vi "MultiFileGraphChoose.vi"(10 "Relationship":T2, 11 "MultiPlot":T1) -> (3 "XYDataOut":cluster{"X":dbl[], "Y":dbl[]}[](array[cluster]))   [LabVIEW 2012]
doc: "读取多个文件中的某一个波形。\n\nname：蒋松\nEmail：jiangsong@outlook.com"
panel:
  out "error out":errorcluster
  in  "error in (no error)":errorcluster
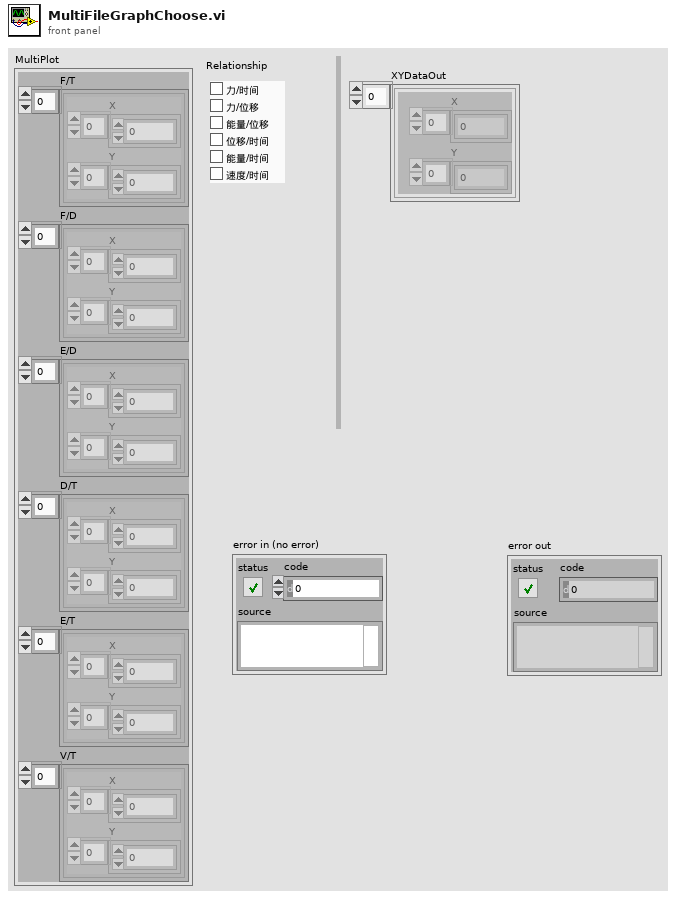
[diagram p1: front panel]
types:
  T1 = cluster{"F/T":cluster{"X":dbl[], "Y":dbl[]}[], "F/D":cluster{"X":dbl[], "Y":dbl[]}[], "E/D":cluster{"X":dbl[], "Y":dbl[]}[], "D/T":cluster{"X":dbl[], "Y":dbl[]}[], "E/T":cluster{"X":dbl[], "Y":dbl[]}[], "V/T":cluster{"X":dbl[], "Y":dbl[]}[]}
  T2 = cluster{"F/T":bool, "F/D":bool, "E/D":bool, "D/T":bool, "E/T":bool, "V/T":bool}
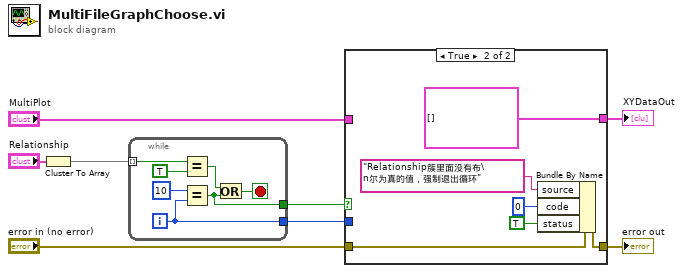
[diagram p0: block diagram]
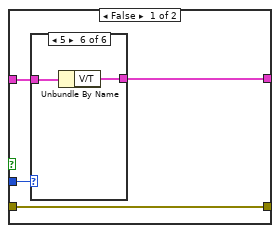
[diagram p2: hidden frame]
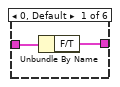
[diagram p3: hidden frame]
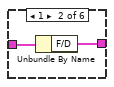
[diagram p4: hidden frame]
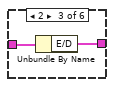
[diagram p5: hidden frame]
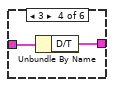
[diagram p6: hidden frame]
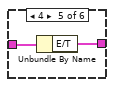
[diagram p7: hidden frame]
diagram:
  n1 = Cluster To Array(cluster="Relationship") -> (array=w7:bool[])
  n2 = while {
    tunnel: w7 -> [w15] mode=indexing
    tunnel: [w11] -> w5
    tunnel: [w9] -> w6
    i -> [w11]
    stop <- w13 stop-if-true
    n3 = Equal?(x=w15, y=TRUE) -> (x = y?=w12:bool)
    n4 = Equal?(x=10, y=w11) -> (x = y?=w9:bool)
    n5 = Or(x=w12, y=w9) -> (x .or. y?=w13:bool)
  }
  n6 = case shown="True" w6 {
    tunnel: w5 -> [w19 _]
    tunnel: "MultiPlot" -> [w18 _]
    tunnel: [w17 cluster{"X":dbl[], "Y":dbl[]}[] [] ("V/T")] -> w3
    tunnel: "error in (no error)" -> [w16 w36]
    tunnel: [w16 w35] -> w1
    frame False {
      n7 = case shown="5" w19 {
        tunnel: w18 -> [w21 w23 w25 w27 w29 w31]
        tunnel: [w20 w22 w24 w26 w28 w30] -> w17
        frame 0, Default {
          n8 = Unbundle By Name(w21) -> ("F/T"=w20:cluster{"X":dbl[], "Y":dbl[]}[])
        }
        frame 1 {
          n9 = Unbundle By Name(w23) -> ("F/D"=w22:cluster{"X":dbl[], "Y":dbl[]}[])
        }
        frame 2 {
          n10 = Unbundle By Name(w25) -> ("E/D"=w24:cluster{"X":dbl[], "Y":dbl[]}[])
        }
        frame 3 {
          n11 = Unbundle By Name(w27) -> ("D/T"=w26:cluster{"X":dbl[], "Y":dbl[]}[])
        }
        frame 4 {
          n12 = Unbundle By Name(w29) -> ("E/T"=w28:cluster{"X":dbl[], "Y":dbl[]}[])
        }
        frame 5 {
          n13 = Unbundle By Name(w31) -> ("V/T"=w30:cluster{"X":dbl[], "Y":dbl[]}[])
        }
      }
    }
    frame True {
      n14 = Bundle By Name(cluster=w36, "source"="Relationship簇里面没有布\n尔为真的值，强制退出循环", "code"=0, "status"=TRUE) -> (w35:errorcluster)
    }
  }
  "error out" <- w1
  "XYDataOut" <- w3
